vi "SimusinWaveform.vi"(2 "canal":i32, 5 "error in (no error)":errorcluster) -> (16 "output waveform":waveform(sgl), 19 "error out":errorcluster)   [LabVIEW 2012, in "SimusinClient.lvlib"]
uses:
  SimusinClient.lvlib
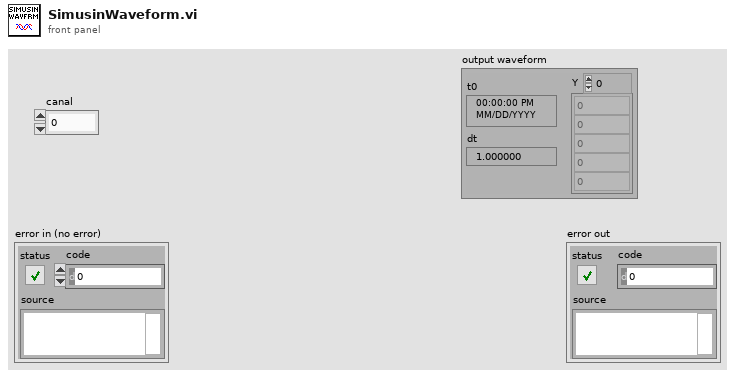
[diagram p1: front panel]
types:
  T1 = typedef "Tipo_PacoteModuloCRIO.ctl" = cluster{"modulo":T2, "sinais":cluster{"dados":sgl[]}[], "numBloco":i32}
  T2 = typedef "Tipo_moduloCRIO.ctl" = cluster{"nome":string, "modelo":string, "slot":i32, "numCanais":i32, "canaisInativos":i32[], "sensores":string[], "TaxaAquisicao":dbl}
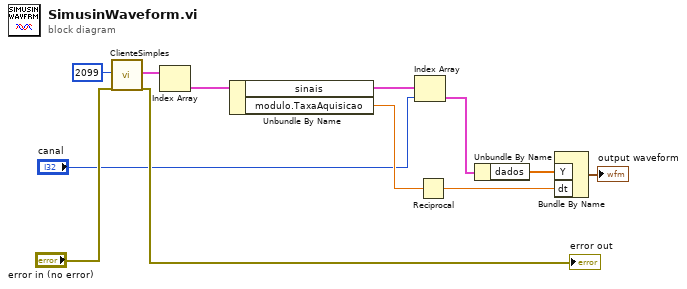
[diagram p0: block diagram]
diagram:
  n1 = call "ClienteSimples.vi"("remote port"=u16 2099, "error in (no error)"="error in (no error)") -> ("value"=w5:T1[], "error out"=→"error out":errorcluster)  [unwired: 16 in]
  n2 = Index Array(array=w5) -> (element=w11:T1)  [unwired: 1 in]
  n3 = Unbundle By Name(w11) -> ("sinais"=w10:cluster{"dados":sgl[]}[], "modulo.TaxaAquisicao"=w8:dbl)
  n4 = Index Array(array=w10, index="canal") -> (element=w9:cluster{"dados":sgl[]})
  n5 = Reciprocal(x=w8) -> (1/x=w6:dbl)
  n6 = Unbundle By Name(w9) -> ("dados"=w7:sgl[])
  n7 = Bundle By Name("Y"=w7, "dt"=w6) -> (→"output waveform":waveform(sgl))  [unwired: 1 in]
